vi "Insert Multiple Events.vi"(4 "Insert all? (T)":bool=TRUE, 5 "Insert Selected?":bool[](array[boolean]), 6 "Events to Insert":string[](array[string]), 7 "Event queue in":string[](array[string])) -> (3 "Event queue out":string[](array[string]))   [LabVIEW 2014]
doc: "Inserts an event or list of events into the event queue. Inserting is conditional based on the 'Insert' control."
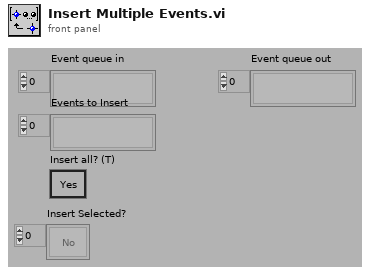
[diagram p1: front panel]
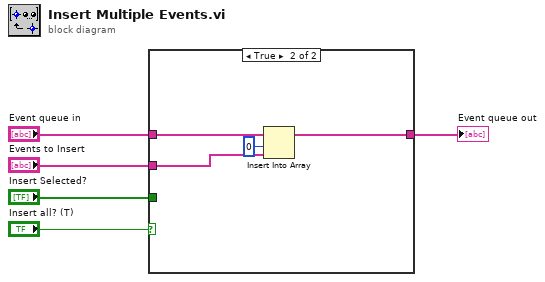
[diagram p0: block diagram]
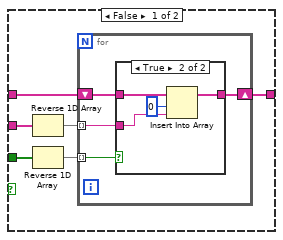
[diagram p2: hidden frame]
diagram:
  n1 = case shown="True" "Insert all? (T)" {
    tunnel: "Event queue in" -> [w11 w24]
    tunnel: [w10 w21] -> w4
    tunnel: "Insert Selected?" -> [w7 _]
    tunnel: "Events to Insert" -> [w9 w22]
    frame False {
      n2 = Reverse 1D Array(array=w9) -> (reversed array=w8:string[])
      n3 = Reverse 1D Array(array=w7) -> (reversed array=w6:bool[])
      n4 = for {
        tunnel: w8 -> [w15] mode=indexing
        tunnel: w6 -> [w12] mode=indexing
        shift-right: [w13] -> w10
        shift-left: w11 -> [w14]
        n5 = case shown="True" w12 {
          tunnel: w15 -> [_ w19]
          tunnel: [w16 w18] -> w13
          tunnel: w14 -> [w16 w20]
          frame False {
          }
          frame True {
            n6 = Insert Into Array(array=w20, index=0 ("Index"), new element=w19) -> (w18:string[])
          }
        }
      }
    }
    frame True {
      n7 = Insert Into Array(array=w24, index=0 ("Index"), new element=w22) -> (w21:string[])
    }
  }
  "Event queue out" <- w4
